vi "InitialSlope.vi"(3 "H (x-axis)":dbl[](array[numeric]), 5 "B (y-axis)":dbl[](array[numeric])) -> (0 "Initial Slope":dbl, 1 "all gradients":dbl[](array[numeric]), 2 "Index of value closest to 0":i32)   [LabVIEW 2019]
panel:
  out "error out":errorcluster
  out "First x value below 0":dbl
  out "Index of First x value below 0":i32
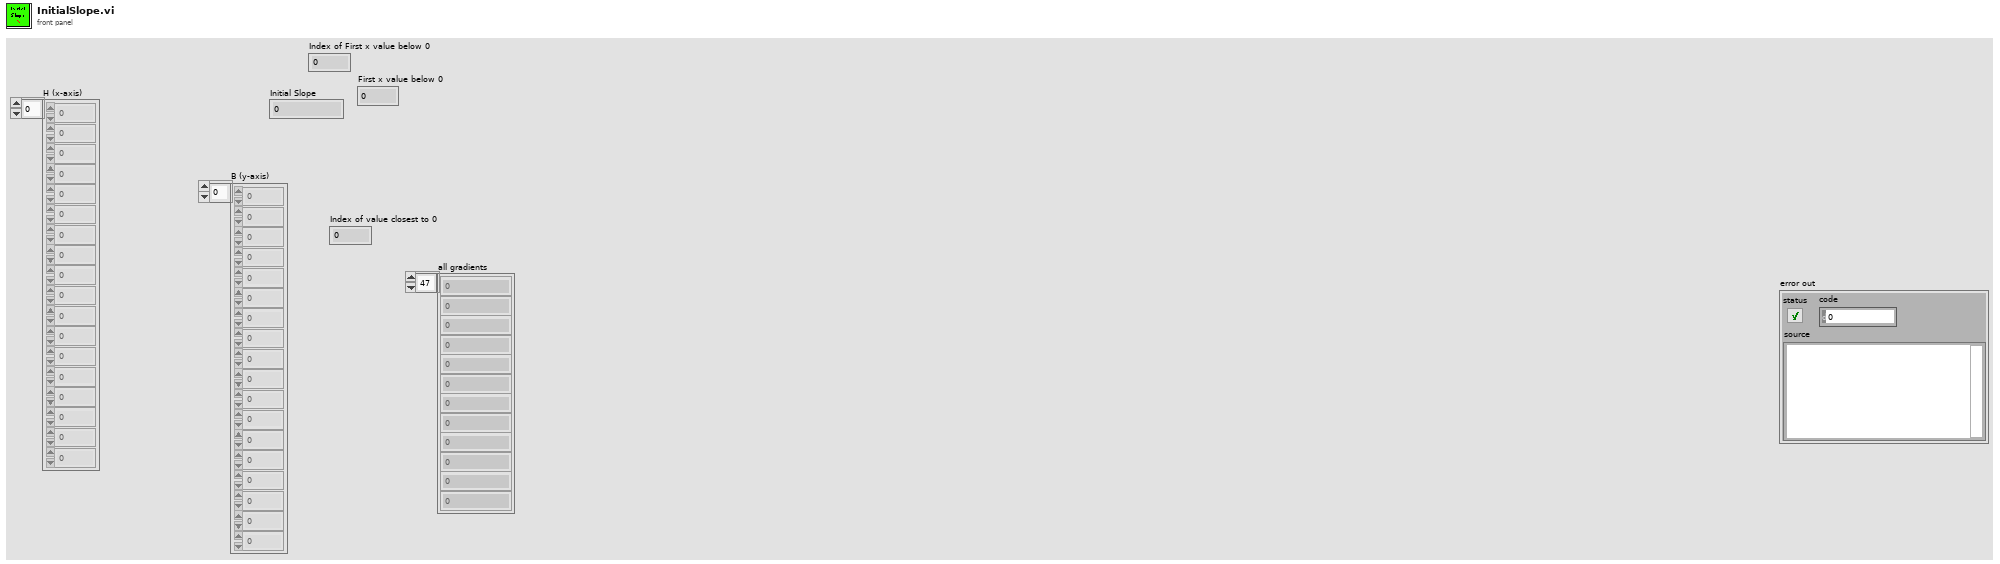
[diagram p1: front panel]
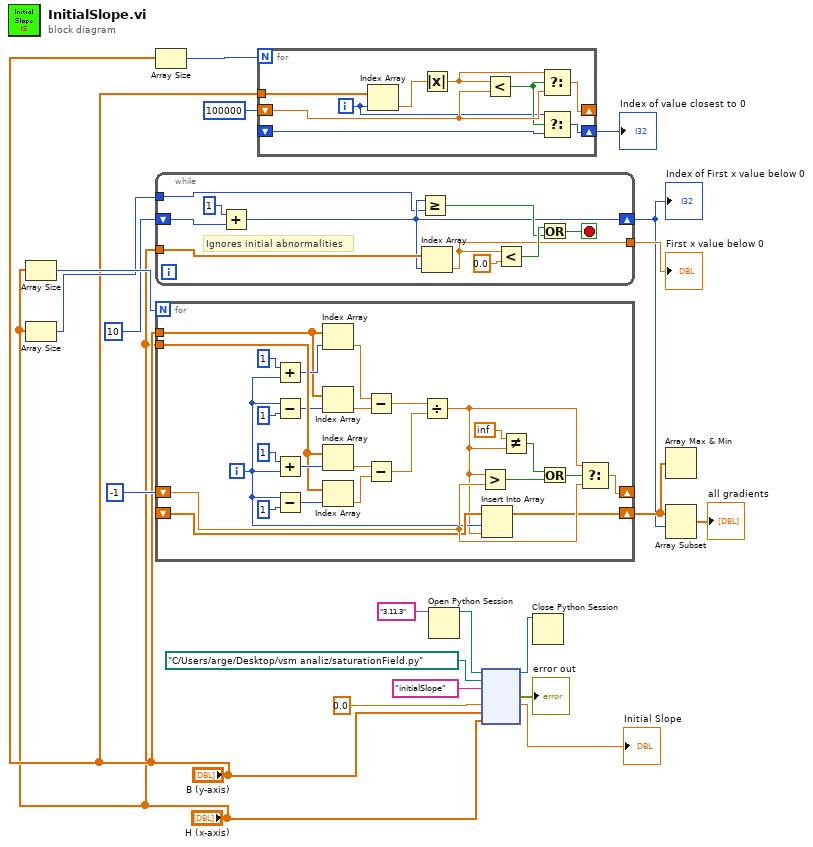
[diagram p0: block diagram]
diagram:
  n1 = Array Size(array="H (x-axis)") -> (size(s)=w18:i32)
  n2 = Array Size(array="H (x-axis)") -> (size(s)=w15:i32)
  n3 = Array Size(array="B (y-axis)") -> (size(s)=w21:i32)
  n4 = while {
    tunnel: "H (x-axis)" -> [w31]
    shift-right: [w24] -> w12
    shift-left: 10 -> [w28]
    tunnel: w15 -> [w23]
    tunnel: [w22] -> w14
    stop <- w26 stop-if-true
    # "Ignores initial abnormalities"
    n5 = Add(x=1, y=w28) -> (x+y=w24:i32)
    n6 = Greater Or Equal?(x=w24, y=w23) -> (x >= y?=w25:bool)
    n7 = Index Array(array=w31, index=w24) -> (element=w22:dbl)
    n8 = Less?(x=w22, y=0.0) -> (x < y?=w29:bool)
    n9 = Or(x=w29, y=w25) -> (x .or. y?=w26:bool)
  }
  "Index of First x value below 0" <- w12
  "First x value below 0" <- w14
  n10 = for {
    N: w18 -> [_]
    tunnel: "H (x-axis)" -> [w55]
    tunnel: "B (y-axis)" -> [w50]
    shift-right: [w43] -> _
    shift-left: -1 -> [w44]
    shift-right: [w40] -> w13
    shift-left: _ -> [w39]
    i -> [w37]
    n11 = Add(x=1 ("y"), y=w37) -> (x+y=w52:i32)
    n12 = Subtract(x=w37, y=1) -> (x-y=w53:i32)
    n13 = Add(x=1 ("y"), y=w37) -> (x+y=w56:i32)
    n14 = Subtract(x=w37, y=1) -> (x-y=w57:i32)
    n15 = Index Array(array=w50, index=w52) -> (element=w47:dbl)
    n16 = Index Array(array=w50, index=w53) -> (element=w46:dbl)
    n17 = Index Array(array=w55, index=w56) -> (element=w48:dbl)
    n18 = Index Array(array=w55, index=w57) -> (element=w49:dbl)
    n19 = Subtract(x=w47, y=w46) -> (x-y=w41:dbl)
    n20 = Subtract(x=w48, y=w49) -> (x-y=w42:dbl)
    n21 = Divide(x=w41, y=w42) -> (x/y=w34:dbl)
    n22 = Greater?(x=w34, y=w44) -> (0:w45:bool)
    n23 = Insert Into Array(array=w39, index=w37, new element=w34) -> (w40:dbl[])
    n24 = Not Equal?(x=inf, y=w34) -> (x != y?=w32:bool)
    n25 = Or(x=w32, y=w45) -> (x .or. y?=w33:bool)
    n26 = Select(t=w34, s=w33, f=w44) -> (s? t:f=w43:dbl)
  }
  n27 = for {
    N: w21 -> [_]
    tunnel: "B (y-axis)" -> [w66]
    shift-right: [w64] -> _
    shift-left: 100000 -> [w65]
    shift-right: [w60] -> w19
    shift-left: _ -> [w61]
    i -> [w62]
    n28 = Index Array(array=w66, index=w62) -> (element=w59:dbl)
    n29 = Absolute Value(x=w59) -> (abs(x)=w58:dbl)
    n30 = Less?(x=w58, y=w65) -> (x < y?=w63:bool)
    n31 = Select(t=w58, s=w63, f=w65) -> (s? t:f=w64:dbl)
    n32 = Select(t=w62, s=w63, f=w61) -> (s? t:f=w60:i32)
  }
  "Index of value closest to 0" <- w19
  n33 = Open Python Session(python version="3.11.3" ("Python version")) -> (session out=w6:refnum<k35>)  [unwired: 2 in, 1 out]
  n34 = node(w6, path "C:/Users/arge/Desktop/vsm analiz/saturationField.py" ("module path"), "initialSlope" ("function name"), 0.0, "B (y-axis)", "H (x-axis)") -> (w5:refnum<k35>, →"error out":errorcluster, →"Initial Slope":dbl)  [unwired: 3 in, 2 out]
  n35 = Close Python Session(session in=w5) -> ()  [unwired: 1 in, 1 out]
  n36 = Array Max & Min(array=w13) -> ()  [unwired: 4 out]
  n37 = Array Subset(array=w13, index=w12) -> (→"all gradients":dbl[])  [unwired: 1 in]
